vi "OE1022D_Configure Equation.vi"(7 "OE1022D_Configure Equation":T1={"A"=0, "B"=18, "C"=19, "E"=1, "C1"=0.0, "C2"=0.0, "Channel"=1} {"Channel" items=["A"=1, "B"=2]; "C2" min=-10.0 max=10.0 format="%.3f"; "C1" min=-10.0 max=10.0 format="%.3f"; "E" items=["1"=1, "2"=2, "3"=3, "4"=4]; "C" items=["R", "X", "Y", "Theta", "Rh1", "Xh1", "Yh1", "Theta h1", "Rh2", "Xh2", "Yh2", "Theta h2", "Noise", "A1", "A2", "A3", "A4", "Freq", "C1", "C2"]; "B" items=["R", "X", "Y", "Theta", "Rh1", "Xh1", "Yh1", "Theta h1", "Rh2", "Xh2", "Yh2", "Theta h2", "Noise", "A1", "A2", "A3", "A4", "Freq", "C1", "C2"]; "A" items=["R", "X", "Y", "Theta", "Rh1", "Xh1", "Yh1", "Theta h1", "Rh2", "Xh2", "Yh2", "Theta h2", "Noise", "A1", "A2", "A3", "A4", "Freq", "C1", "C2"]}, 8 "Error in (no error)":errorcluster caption="error out（no error）", 9 "Remote Mode":u16(ring) items=["USB", "RS232", "GPIB"], 11 "VISA resource name":refnum<visa-resource-name>) -> (0 "Error out":errorcluster caption="error out", 1 "Output String":string, 3 "VISA resource  out":refnum<visa-resource-name>)   [LabVIEW 2011]
panel:
  # "X"
  # "E             ="
  # "______________________________________________________"
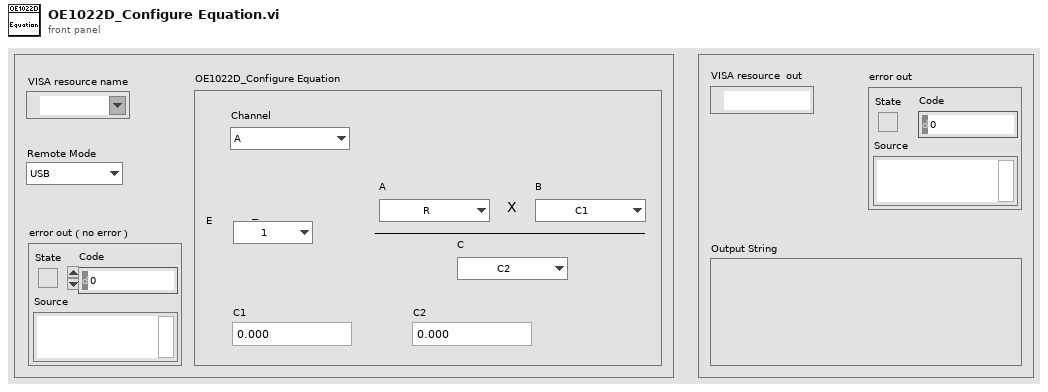
[diagram p1: front panel]
types:
  T1 = cluster{"A":u16, "B":u16, "C":u16, "E":u16, "C1":dbl, "C2":dbl, "Channel":u16}
  T2 = enum16{"ISRC", "IGND", "ICPL", "ILIN", "PHAS", "FMOD", "RSLP", "FREQ", "SWPT", "SLLM", "SULM", "SSLL", "SSLG", "STLM", "SWRM", "IRNG", "SENS", "RMOD", "OFLT", "OFSL", "SYNC", "DMOD", "HARM", "DARB", "SWVT", "SLVL", "SVLL", "SVUL", "SVSL", "SVSG", "SVTM", "SVRM", "RALL", "SNAP", "OUTP", "OAUX", "COUT", "CAUX", "COFP", "CEXP", "FPOP", "OEXP", "*IDN", "*RST", "OVLD", "INOV", "GNOV", "*PLL", "SSET", "RSET", "AGAN", "APHS", "ARSV", "ASCL", "EQCD", "EQCS", "SPED", "SRAT", "SLEN", "SSLE", "STRG", "SPRM", "STRD", "PAUS", "REST", "SPTS", "TRCA", "TEMP", "RSTU", "IHNZ", "DEQU", "SADD", "ARNG", "CSPE", "ISRCD", "IGNDD", "ICPLD", "ILIND", "PHASD", "FMODD", "RSLPD", "FREQD", "SWPTD", "SLLMD", "SULMD", "SSLLD", "SSLGD", "STLMD", "SWRMD", "SENSD", "RMODD", "OFLTD", "OFSLD", "SYNCD", "HARMD", "EQCDD", "EQCSD", "SNAPD", "OUTPD", "SWVTD", "SLVLD", "SVLLD", "SVULD", "SVSLD", "SVSGD", "SVTMD", "SVRMD", "SVDCD", "ARSVD", "AGAND", "APHSD", "ASCLD", "FPOPD", "CAUXD", "OEXPD", "SPEDD", "SRATD", "SLEND", "SSLED", "STRGD", "SPRMD", "STRDD", "PAUSD", "RESTD", "SPTSD", "TRCAD", "*IDND", "*RSTD", "INOVD", "GNOVD", "*PLLD", "SSETD", "RSETD"}
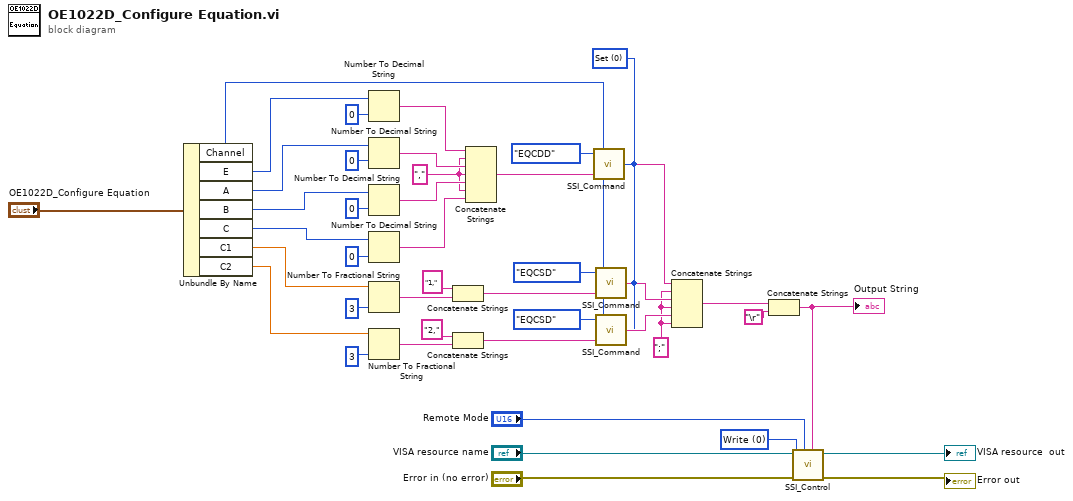
[diagram p0: block diagram]
diagram:
  w4 = ";" ("替换字符串(\"\")")
  w6 = u16 0 items=["Set", "Query"] ("Opera")
  w7 = "," ("替换字符串(\"\")")
  w42 = u16 0 items=["Write", "Read"] ("Control")
  n1 = Unbundle By Name("OE1022D_Configure Equation") -> ("Channel"=w1:u16, "E"=w18:u16, "A"=w17:u16, "B"=w16:u16, "C"=w15:u16, "C1"=w14:dbl, "C2"=w13:dbl)
  n2 = Number To Decimal String(number=w18, width (-)=i16 0 ("精度(6)")) -> (decimal integer string=w12:string)
  n3 = Number To Decimal String(number=w17, width (-)=i16 0 ("宽度(-)")) -> (decimal integer string=w11:string)
  n4 = Number To Decimal String(number=w16, width (-)=i16 0 ("宽度(-)")) -> (decimal integer string=w10:string)
  n5 = Number To Decimal String(number=w15, width (-)=i16 0 ("宽度(-)")) -> (decimal integer string=w9:string)
  n6 = Number To Fractional String(number=w14, precision (6)=i16 3 ("宽度(-)")) -> (F-format string=w23:string)  [unwired: 2 in]
  n7 = Number To Fractional String(number=w13, precision (6)=i16 3 ("宽度(-)")) -> (F-format string=w22:string)  [unwired: 2 in]
  n8 = Concatenate Strings("1," ("替换字符串(\"\")"), w23) -> (w24:string)
  n9 = Concatenate Strings("2," ("替换字符串(\"\")"), w22) -> (w21:string)
  n10 = Concatenate Strings(w12, w7, w11, w7, w10, w7, w9) -> (w8:string)
  n11 = call "SSI_Command.vi"("Opera"=w6, "Paramter"=w8, "channel"=w1, "Command Type"=T2."EQCDD") -> ("Output string"=w5:string)
  n12 = call "SSI_Command.vi"("Opera"=w6, "Paramter"=w24, "channel"=w1, "Command Type"=T2."EQCSD") -> ("Output string"=w34:string)
  n13 = call "SSI_Command.vi"("Opera"=w6, "Paramter"=w21, "channel"=w1, "Command Type"=T2."EQCSD") -> ("Output string"=w25:string)
  n14 = Concatenate Strings(w5, w4, w34, w4, w25, w4) -> (w2:string)
  n15 = Concatenate Strings(w2, "\r") -> (w37:string)
  "Output String" <- w37
  n16 = call "SSI_Control.vi"("Write Buffer"=w37, "Remote Mode"="Remote Mode", "Error in (no error)"="Error in (no error)", "Control"=w42, "VISA resource name"="VISA resource name") -> ("Error out"=→"Error out":errorcluster, "VISA resource  out"=→"VISA resource  out":refnum<visa-resource-name>)  [unwired: 3 in, 2 out]
